vi "Current Path.vi"() -> ()   [LabVIEW 2017, in "Pure Pursuit.lvlib"]
uses:
  Pure Pursuit.lvlib
panel:
  in  "Current Path":cluster{"X Out":dbl[], "Y Out":dbl[]}
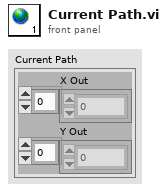
[diagram p1: front panel]
diagram:
